vi "New Footer From Document.vi"(7 "xwpfHeader in":refnum<class "xwpfHeader_Footer.lvclass">, 8 "error in (no error)":errorcluster, 11 "Footer Ref":refnum<k24>) -> (0 "error out":errorcluster, 3 "xwpfHeader out":refnum<class "xwpfHeader_Footer.lvclass">)   [LabVIEW 2017, in "Word_Specific.lvlib" / "xwpfHeader_Footer.lvclass"]
uses:
  xwpfHeader_Footer.lvclass
  C:/Users/Neo/Desktop/Dev_Tools_BR/LabVIEW_NPOI/src/lib/NPOI 2.1.1/NPOI.OOXML.dll
  lib/NPOI 2.1.1/NPOI.OOXML.dll
  xwpfHeader_Footer.lvclass/xwpfHeader_Footer.ctl
  xwpfParagraph/xwpfParagraph.lvclass
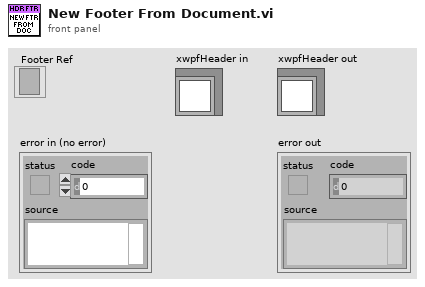
[diagram p1: front panel]
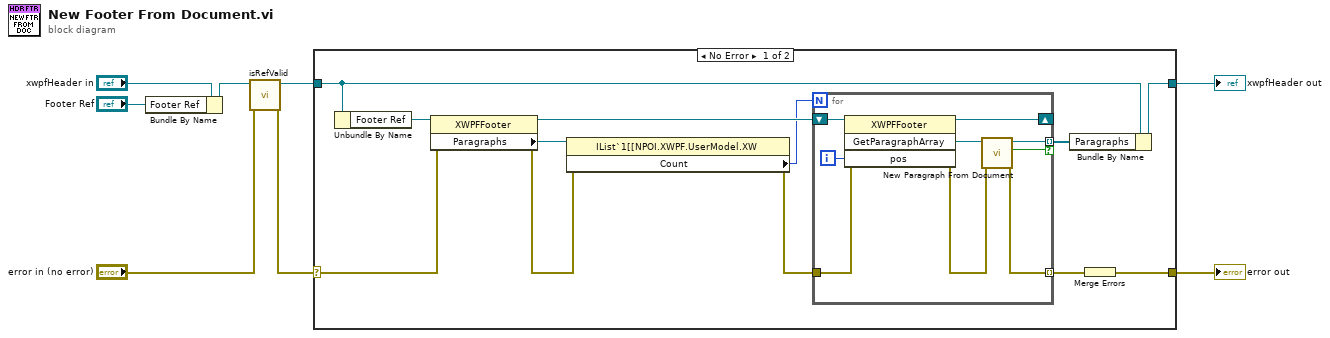
[diagram p0: block diagram]
diagram:
  n1 = Bundle By Name(cluster="xwpfHeader in", "Footer Ref"="Footer Ref") -> (w3:refnum<class "xwpfHeader_Footer.lvclass">)
  n2 = call-dynamic "isRefValid.vi"("error in (no error)"="error in (no error)", "xwpfHeader in"=w3) -> ("error out"=w1:errorcluster, "xwpfHeader out"=w2:refnum<class "xwpfHeader_Footer.lvclass">)  [unwired: 8 in]
  n3 = case shown="No Error" w1 {
    selector: w1 -> [w18 w31]
    tunnel: w2 -> [w19 w30]
    tunnel: [w13 w31] -> w7
    tunnel: [w10 w30] -> w5
    frame No Error {
      n4 = Unbundle By Name(w19) -> ("Footer Ref"=w20:refnum<k24>)
      n5 = property class="XWPFFooter"(reference=w20, error in=w18) -> (reference out=w15:refnum<k24>, error out=w16:errorcluster, "Paragraphs"=w17:refnum<k24>)
      n6 = property class="IList`1[[NPOI.XWPF.UserModel.XW"(reference=w17, error in=w16) -> (error out=w11:errorcluster, "Count"=w12:i32)  [unwired: 1 out]
      n7 = for {
        N: w12 -> [_]
        shift-right: [w26] -> _
        shift-left: w15 -> [w29]
        tunnel: [w23] -> w14 mode=indexing
        tunnel: w11 -> [w27]
        tunnel: [w22] -> w9 mode=indexing if=w21
        i -> [w28]
        n8 = invoke class="XWPFFooter" method="GetParagraphArray"(reference=w29, error in=w27, "pos"=w28) -> (reference out=w26:refnum<k24>, error out=w24:errorcluster, "GetParagraphArray"=w25:refnum<k24>)  [unwired: 1 in, 1 out]
        n9 = call "New Paragraph From Document.vi"("error in (no error)"=w24, "Paragraph Ref"=w25) -> ("error out"=w23:errorcluster, "New Element Found"=w21:bool, "xwpfParagraph out"=w22:refnum<class "xwpfParagraph.lvclass">)  [unwired: 7 in]
      }
      n10 = Bundle By Name(cluster=w19, "Paragraphs"=w9) -> (w10:refnum<class "xwpfHeader_Footer.lvclass">)
      n11 = Merge Errors(w14) -> (w13:errorcluster)
    }
    frame Error {
    }
  }
  "error out" <- w7
  "xwpfHeader out" <- w5
